vi "make_readout_alarm_LCW.vi"(3 "enabled":bool=TRUE, 7 "ref_n_error":refnum<vi>, 8 "time_last_alarm_in":timestamp, 10 "readout_status":bool=TRUE) -> (0 "time_last_alarm_out":timestamp, 2 "alarm_status":u32(colorbox))   [LabVIEW 2019]
panel:
  in  "interval":dbl=600.0
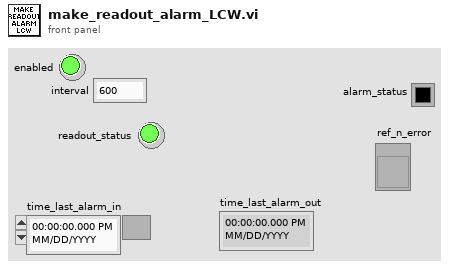
[diagram p1: front panel]
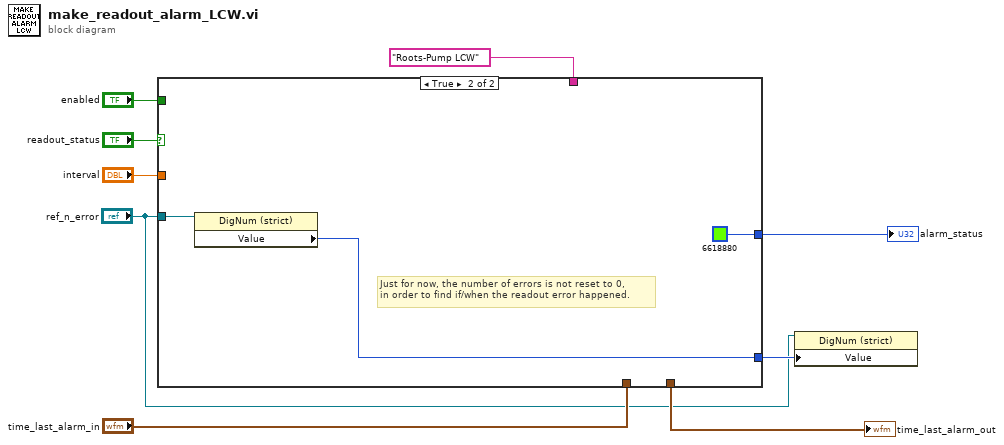
[diagram p0: block diagram]
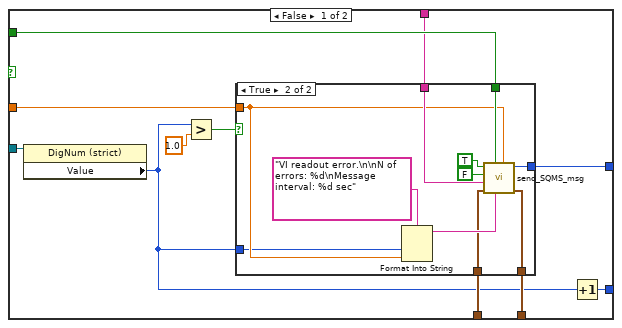
[diagram p2: hidden frame]
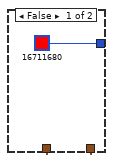
[diagram p3: hidden frame]
diagram:
  n1 = case shown="True" "readout_status" {
    tunnel: "interval" -> [w13 _]
    tunnel: "ref_n_error" -> [w19 w35]
    tunnel: "enabled" -> [w18 _]
    tunnel: "time_last_alarm_in" -> [w17 w37]
    tunnel: "Roots-Pump LCW" ("title") -> [w16 _]
    tunnel: [w15 w37] -> w4
    tunnel: [w14 u32 6618880 ("alarm_status")] -> w3
    tunnel: [w11 w34] -> w2
    frame False {
      n2 = property on="Property Node" class="DigNum (strict)"(reference=w19) -> ("Value"=w10:i8)  [unwired: 1 in, 2 out]
      n3 = Greater?(x=w10, y=1.0) -> (0:w12:bool)
      n4 = case shown="True" w12 {
        tunnel: w18 -> [_ w31]
        tunnel: w17 -> [w22 w30]
        tunnel: w16 -> [_ w29]
        tunnel: [w22 w28] -> w15
        tunnel: [u32 16711680 ("alarm_status") w27] -> w14
        tunnel: w13 -> [_ w24]
        tunnel: w10 -> [_ w23]
        frame False {
        }
        frame True {
          n5 = Format Into String(format string="VI readout error.\n\nN of errors: %d\nMessage interval: %d sec" ("msg"), w23, w24) -> (resulting string=w32:string)  [unwired: 2 in, 1 out]
          n6 = call "send_SQMS_msg.vi"("alarm_interval"=w24, "msg"=w32, "enabled"=w31, "time_last_alarm_in"=w30, "title"=w29, "warning"=FALSE, "error"=TRUE) -> ("time_last_alarm_out"=w28:timestamp, "alarm_status"=w27:u32)  [unwired: 2 in, 1 out]
        }
      }
      n7 = Increment(x=w10) -> (x+1=w11:i8)
    }
    frame True {
      # "Just for now, the number of errors is not reset to 0,\nin order to find if/when the readout error happened."
      n8 = property on="Property Node" class="DigNum (strict)"(reference=w35) -> ("Value"=w34:i8)  [unwired: 1 in, 2 out]
    }
  }
  "time_last_alarm_out" <- w4
  "alarm_status" <- w3
  n9 = property on="Property Node" class="DigNum (strict)"(reference="ref_n_error", "Value"=w2) -> ()  [unwired: 1 in, 2 out]
